vi "W_inv__transfer_X.vi"(4 "x":dbl format="%#_13g") -> (1 "y":dbl)   [LabVIEW 2015]
panel:
  out "x*y 2":dbl[](array[numeric])
  out "Error (mm)":dbl[][](graph)
  out "x*y":dbl[](array[numeric])
  out "array w/ subset deleted":dbl[](array[numeric])
  in  "Wn":dbl[](array[numeric])=[1.0, -2.58482411682536, 2.53656993452636, -1.23969117603537, 0.311595918708408, -0.0208467121118959] format="%#_13g"
  in  "Wd":dbl[](array[numeric])=[1.0, -3.33482411682431, 4.30572826538785, -2.66569311478873, 0.779063032726811, -0.0833868484477247] format="%#_13g"
  out "yk chain":dbl[](array[numeric])
  out "xk chain":dbl[](array[numeric])
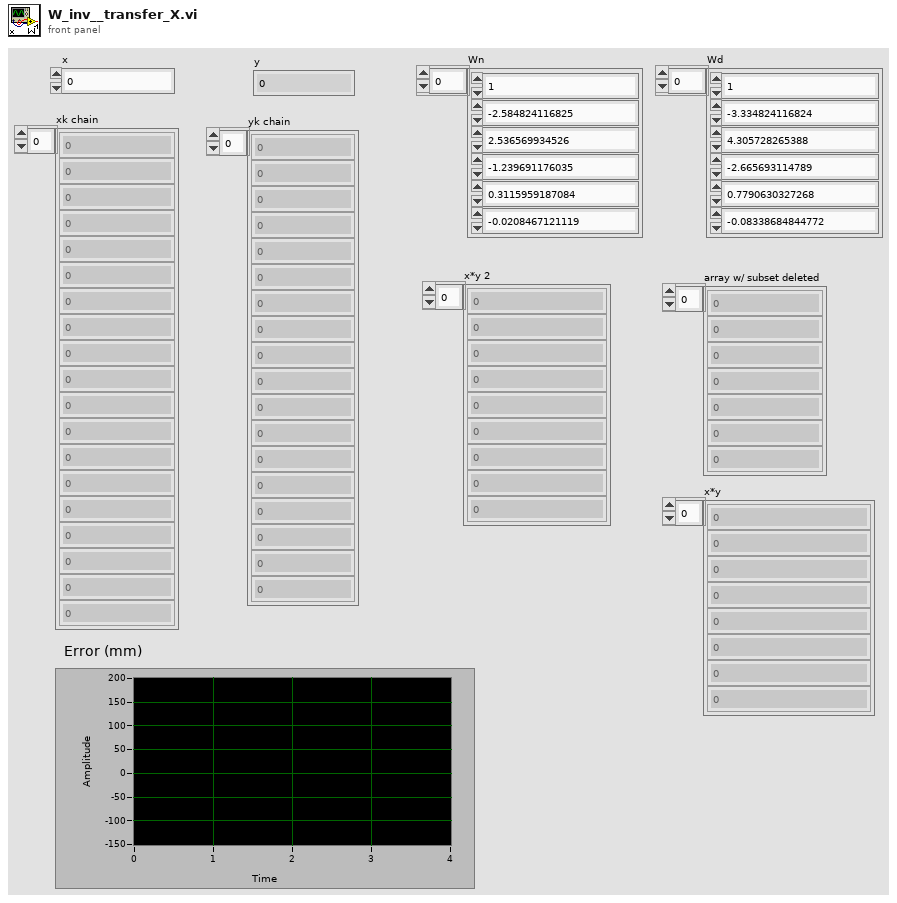
[diagram p1: front panel]
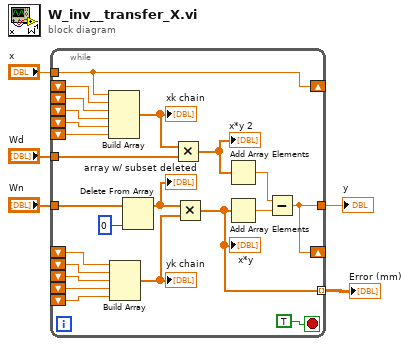
[diagram p0: block diagram]
diagram:
  n1 = while {
    tunnel: [w21] -> w4
    tunnel: "x" -> [w23]
    tunnel: "Wn" -> [w17]
    tunnel: "Wd" -> [w18]
    shift-right: [w23] -> _
    shift-left: _ -> [w22]
    shift-right: [w21] -> _
    shift-left: _ -> [w16]
    shift-left: _ -> [w14]
    shift-left: _ -> [w13]
    shift-left: _ -> [w12]
    shift-left: _ -> [w11]
    shift-left: _ -> [w10]
    shift-left: _ -> [w9]
    tunnel: [w8] -> w5 mode=indexing
    shift-left: _ -> [w7]
    shift-left: _ -> [w6]
    stop <- TRUE stop-if-true
    n2 = Build Array(w23, w22, w11, w10, w9, w7) -> (w19:dbl[])
    "xk chain" <- w19
    n3 = Build Array(w16, w14, w13, w12, w6) -> (w15:dbl[])
    "yk chain" <- w15
    n4 = Delete From Array(array=w17, index=0) -> (array with subset deleted=w26:dbl[])  [unwired: 1 in, 1 out]
    "array w/ subset deleted" <- w26
    n5 = Multiply(x=w19, y=w18) -> (x*y=w28:dbl[])
    "x*y 2" <- w28
    n6 = Multiply(x=w26, y=w15) -> (x*y=w8:dbl[])
    "x*y" <- w8
    n7 = Add Array Elements(numeric array=w28) -> (sum=w25:dbl)
    n8 = Add Array Elements(numeric array=w8) -> (sum=w24:dbl)
    n9 = Subtract(x=w25, y=w24) -> (x-y=w21:dbl)
  }
  "y" <- w4
  "Error (mm)" <- w5
